vi "setupCam.vi"(2 "Error IN":errorcluster, 3 "Camera Handle":u32) -> (0 "error out":errorcluster)   [LabVIEW 2020]
panel:
  out "ADC Speed":i32
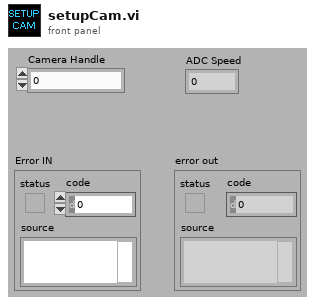
[diagram p1: front panel]
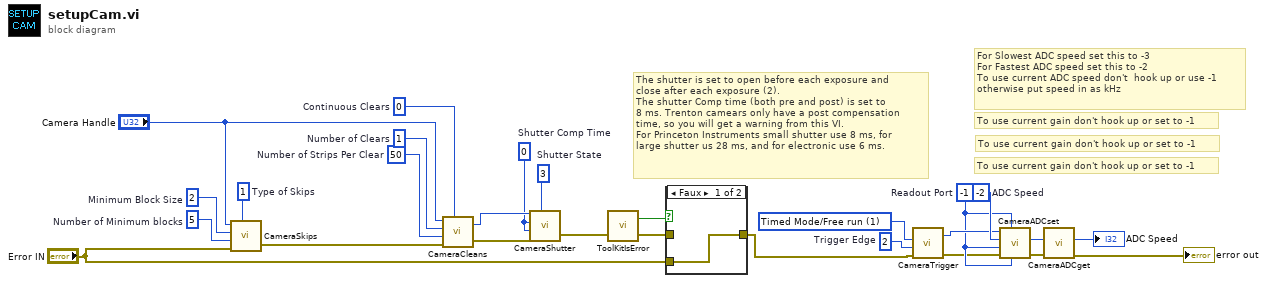
[diagram p0: block diagram]
diagram:
  w12 = -2  # ADC Speed
  w9 = -1  # Readout Port
  w8 = u32 1 items=["N/A", "Timed Mode/Free run", "Trigger First (only PM)", "Strobed/Ext Sync", "Bulb Mode (PM only)", "Variable Timed mode (PM only)", "Flash Mode (only some PM)"] ("Timing Mode")
  w3 = u32 2  # Trigger Edge
  w17 = u32 1  # Type of Skips
  w16 = u32 5  # Number of Minimum blocks
  w15 = u32 2  # Minimum Block Size
  w18 = u32 3  # Shutter State
  w19 = u32 0  # Shutter Comp Time
  w24 = u32 1  # Number of Clears
  w25 = u32 50  # Number of Strips Per Clear
  w23 = u32 0  # Continuous Clears
  # "To use current gain don't hook up or set to -1"
  # "To use current gain don't hook up or set to -1"
  # "To use current gain don't hook up or set to -1"
  # "For Slowest ADC speed set this to -3\nFor Fastest ADC speed set this to -2\nTo use current ADC speed don't  hook up or use -1\notherwise put speed in as kHz"
  # "The shutter is set to open before each exposure and\nclose after each exposure (2).\nThe shutter Comp time (both pre and post) is set to \n8 ms. Trenton camears only have a post compensation \ntime, so you will get a warning from this VI.\nFor Princeton Instruments small shutter use 8 ms, for \nlarge shutter us 28 ms, and for electronic use 6 ms."
  n1 = call <userlib>:"CameraSkips.vi"("Camera Handle"="Camera Handle", "Minimum Block Size"=w15, "Number of Minimum blocks"=w16, "error in"="Error IN", "Type of Skips"=w17) -> ("error out"=w2:errorcluster)  [unwired: 1 out]
  n2 = call <userlib>:"CameraCleans.vi"("Camera Handle"="Camera Handle", "Number of Clears"=w24, "Number of Strips Per Clear"=w25, "error in"=w2, "Continuous Clears"=w23) -> ("Camera Handle"=w21:u32, "error out"=w22:errorcluster)
  n3 = call <userlib>:"CameraShutter.vi"("Camera Handle"=w21, "Shutter Comp Time: Pre Open"=w19, "Shutter Comp Time: Post Open"=w19, "error in"=w22, "Shutter State"=w18) -> ("error out"=w20:errorcluster)  [unwired: 1 out]
  n4 = call <userlib>:"ToolKitIsError.vi"("error in"=w20) -> ("error out"=w26:errorcluster, "Error Flag"=w27:bool)  [unwired: 1 in]
  n5 = case shown="Faux" w27 {
    tunnel: w26 -> [_ w29]
    tunnel: [w28 w29] -> w5
    tunnel: "Error IN" -> [w28 _]
    frame False {
    }
    frame True {
    }
  }
  n6 = call <userlib>:"CameraTrigger.vi"("error in"=w5, "Trigger Edge"=w3, "Timing Mode"=w8) -> ("error out"=w6:errorcluster, "Camera Handle"=w10:u32)  [unwired: 1 in]
  n7 = call <userlib>:"CameraADCset.vi"("ADC offset"=w9, "Read Out port"=w9, "error in (no error)"=w6, "ADC Gain"=w9, "ADC Speed"=w12, "Camera Handle"=w10) -> ("error out"=w7:errorcluster, "Camera Handle"=w11:u32)
  n8 = call <userlib>:"CameraADCget.vi"("Camera handle"=w11, "error in (no error)"=w7) -> ("ADC Speed"=→"ADC Speed":i32, "error out"=→"error out":errorcluster)  [unwired: 6 out]
